vi "App Data Directory.vi"(8 "error in (no error)":errorcluster) -> (0 "error out":errorcluster, 3 "App Data Directory":path)   [LabVIEW 2020, in "MacroAssert.lvlib"]
uses:
  MacroAssert.lvlib
  <userlib>/_OpenG.lib/file/file.llb/openg_file.lvlib
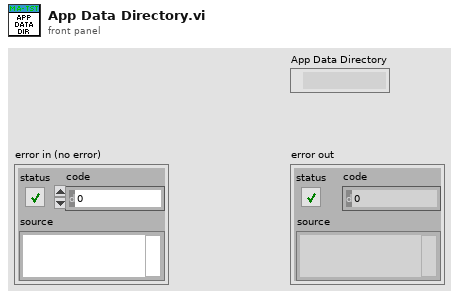
[diagram p1: front panel]
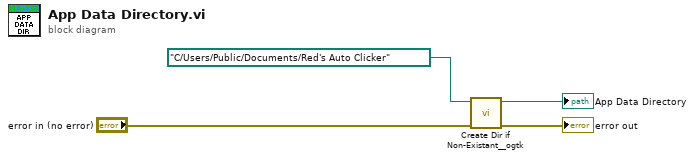
[diagram p0: block diagram]
diagram:
  n1 = call <userlib>:"Create Dir if Non-Existant__ogtk.vi"("error in (no error)"="error in (no error)", "Directory Path"=path "C:/Users/Public/Documents/Red's Auto Clicker") -> ("error out"=→"error out":errorcluster, "dup Directory Path"=→"App Data Directory":path)  [unwired: 7 in, 1 out]
